vi "server.Send Request (Batch Sync).vi"(6 "Timeout (-1)":i32=-1, 8 "error in (no error)":errorcluster, 10 "JSON Request String":string[](array[string]), 11 "JSONRPC Server in":refnum<class "JSONRPC Server.lvclass">) -> (0 "error out":errorcluster, 2 "JSON Response String":string[](array[string]), 3 "JSONRPC Server out":refnum<class "JSONRPC Server.lvclass">)   [LabVIEW 2016, in "JSONRPC Server.lvclass"]
uses:
  JSONRPC Server.lvclass
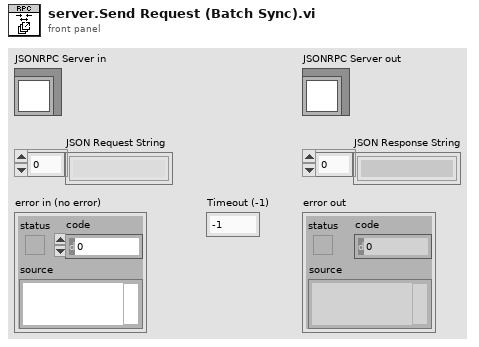
[diagram p1: front panel]
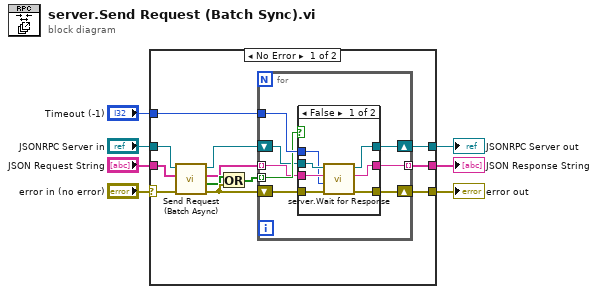
[diagram p0: block diagram]
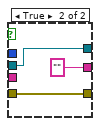
[diagram p2: hidden frame]
diagram:
  n1 = case shown="No Error" "error in (no error)" {
    selector: "error in (no error)" -> [w8 w39]
    tunnel: [w17 w39] -> w6
    tunnel: [w19 w38] -> w4
    tunnel: "JSONRPC Server in" -> [w9 w38]
    tunnel: "JSON Request String" -> [w14 _]
    tunnel: [w18 _] -> w2
    tunnel: "Timeout (-1)" -> [w16 _]
    frame No Error {
      n2 = call "Send Request (Batch Async).vi"("error in (no error)"=w8, "JSON Request String"=w14, "Server in"=w9) -> ("error out"=w13:errorcluster, "notification?"=w12:bool[], "id value"=w11:string[], "Server out"=w10:refnum<class "JSONRPC Server.lvclass">)  [unwired: 5 in]
      n3 = Or(x=w12, y=w13) -> (x .or. y?=w15:bool[])
      n4 = for {
        tunnel: [w26] -> w18 mode=indexing
        tunnel: w16 -> [w24]
        tunnel: w15 -> [w23] mode=indexing
        tunnel: w11 -> [w21] mode=indexing
        shift-right: [w25] -> w17
        shift-left: w13 -> [w22]
        shift-right: [w27] -> w19
        shift-left: w10 -> [w20]
        n5 = case shown="False" w23 {
          tunnel: w20 -> [w34 w37]
          tunnel: [w33 w37] -> w27
          tunnel: w21 -> [w32 _]
          tunnel: w22 -> [w31 w36]
          tunnel: [w30 "" ("JSON Response String")] -> w26
          tunnel: [w29 w36] -> w25
          tunnel: w24 -> [w28 _]
          frame False {
            n6 = call-dynamic "server.Wait for Response.vi"("error in (no error)"=w31, "Timeout (-1)"=w28, "id String"=w32, "JSONRPC Server in"=w34) -> ("error out"=w29:errorcluster, "JSON Response String"=w30:string, "JSONRPC Server out"=w33:refnum<class "JSONRPC Server.lvclass">)  [unwired: 5 in]
          }
          frame True {
          }
        }
      }
    }
    frame Error {
    }
  }
  "error out" <- w6
  "JSONRPC Server out" <- w4
  "JSON Response String" <- w2
